vi "Dictionary Pop Item__ogtk.vi"(8 "error in (no error)":errorcluster, 11 "dictionary":T1) -> (0 "error out":errorcluster, 2 "item":cluster{"key":variant, "value":variant}, 3 "dictionary out":T1)   [LabVIEW 2011]
doc: "Removes and returns a single Item (key - value pair) from the dictionary."
uses:
  Dictionary Object RefNum__ogtk.ctl
  Dictionary Object RefNum - Enum__ogtk.ctl
panel:
  # "Dictionary Pop Item.vi\n\nRemoves and returns a single Item (key - value pair) from the dictionary.\n\nPlease visit http://www.OpenG.org to learn about the\nOpen Source LabVIEW software movement.\n\nNOTICE -- YOU MUST LEAVE THIS NOTICE IN PLACE.  PER THE TERMS OF THE LICENSE BELOW, YOU MAY SUBLICENSE THIS SOFTWARE \nIN ANY WAY THAT DOES NOT CONFLICT WITH THIS LICENSE.\n\n### BSD License (http://www.opensource.org/licenses/bsd-license.php) Begin ###\n \nCopyright (c) 2005, Jim Kring <jim@jimkring.com>\n\nAll rights reserved.\n\nRedistribution and use in source and binary forms, with or without modification, are permitted provided that the following conditions are met:\n\n    * Redistributions of source code must retain the above copyright notice, this list of conditions and the following disclaimer.\n    * Redistributions in binary form must reproduce the above copyright notice, this list of conditions and the following disclaimer in the \n       documentation and/or other materials provided with the distribution.\n    * Neither the name of SciWare, James Kring, Inc., nor the names of its contributors may be used to endorse or promote products derived \n       from this software without specific prior written permission.\n\nTHIS SOFTWARE IS PROVIDED BY THE COPYRIGHT HOLDERS AND CONTRIBUTORS \"AS IS\" AND ANY EXPRESS OR IMPLIED WARRANTIES, \nINCLUDING, BUT NOT LIMITED TO, THE IMPLIED WARRANTIES OF MERCHANTABILITY AND FITNESS FOR A PARTICULAR PURPOSE ARE \nDISCLAIMED. IN NO EVENT SHALL THE COPYRIGHT OWNER OR CONTRIBUTORS BE LIABLE FOR ANY DIRECT, INDIRECT, INCIDENTAL,\n SPECIAL, EXEMPLARY, OR CONSEQUENTIAL DAMAGES (INCLUDING, BUT NOT LIMITED TO, PROCUREMENT OF SUBSTITUTE GOODS OR \nSERVICES; LOSS OF USE, DATA, OR PROFITS; OR BUSINESS INTERRUPTION) HOWEVER CAUSED AND ON ANY THEORY OF LIABILITY, \nWHETHER IN CONTRACT, STRICT LIABILITY, OR TORT (INCLUDING NEGLIGENCE OR OTHERWISE) ARISING IN ANY WAY OUT OF THE USE \nOF THIS SOFTWARE, EVEN IF ADVISED OF THE POSSIBILITY OF SUCH DAMAGE.\n\n### BSD License End ###"
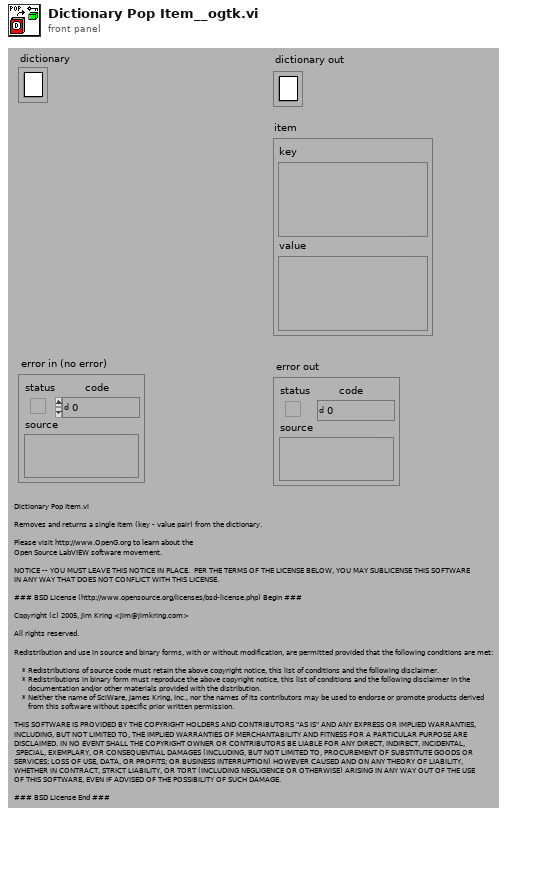
[diagram p1: front panel]
types:
  T1 = typedef "Dictionary Object RefNum__ogtk.ctl" = refnum<k1>
  T2 = typedef "Dictionary Data__ogtk.ctl" = cluster{"keys":variant[], "values":variant[]}
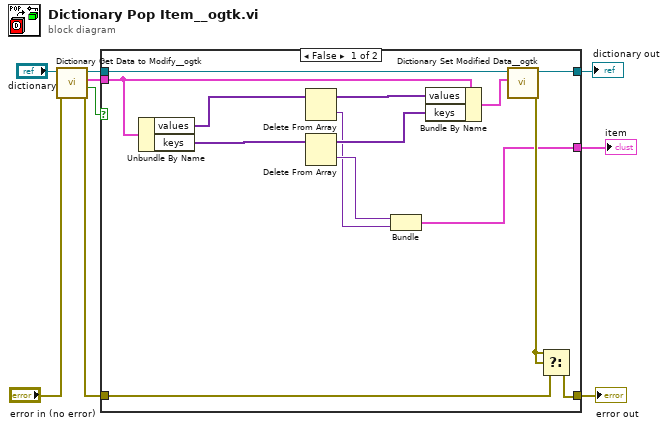
[diagram p0: block diagram]
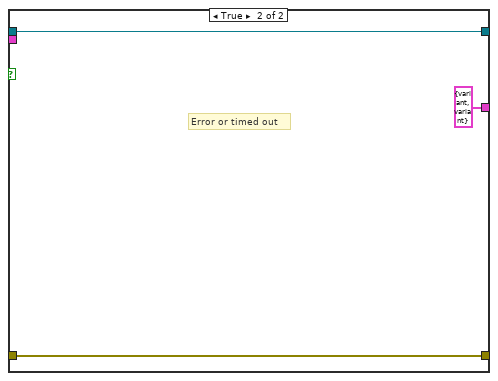
[diagram p2: hidden frame]
diagram:
  n1 = call "Dictionary Get Data to Modify__ogtk.vi"("error in (no error)"="error in (no error)", "Object RefNum"="dictionary") -> ("error out"=w6:errorcluster, "timed out"=w5:bool, "Data out"=w7:T2, "Dup Object RefNum"=w2:T1)  [unwired: 6 in]
  n2 = case shown="False" w5 {
    tunnel: w7 -> [w22 _]
    tunnel: w6 -> [w18 w26]
    tunnel: [w17 w26] -> w8
    tunnel: [w21 w25] -> w3
    tunnel: w2 -> [w20 w25]
    tunnel: [w10 cluster{"Variant":variant, "Variant":variant} {"Variant"=variant, "Variant"=variant}] -> w1
    frame False {
      n3 = Unbundle By Name(w22) -> ("values"=w15:variant[], "keys"=w16:variant[])
      n4 = Delete From Array(array=w15) -> (deleted portion=w11:variant, array with subset deleted=w14:variant[])  [unwired: 2 in]
      n5 = Delete From Array(array=w16) -> (deleted portion=w12:variant, array with subset deleted=w13:variant[])  [unwired: 2 in]
      n6 = Bundle("Variant"=w12, "Variant"=w11) -> (w10:cluster{"Variant":variant, "Variant":variant})  [unwired: 1 in]
      n7 = Bundle By Name(cluster=w22, "values"=w14, "keys"=w13) -> (w23:T2)
      n8 = call "Dictionary Set Modified Data__ogtk.vi"("Data in"=w23, "Object RefNum"=w20) -> ("error out"=w19:errorcluster, "dup Object RefNum"=w21:T1)  [unwired: 8 in]
      n9 = Select(t=w19, s=w19, f=w18) -> (s? t:f=w17:errorcluster)
    }
    frame True {
      # "Error or timed out"
    }
  }
  "error out" <- w8
  "dictionary out" <- w3
  "item" <- w1
